vi "VI Tree.vi"   [LabVIEW 2013, in "Keithley 2000.lvlib"]
doc: "This is the instrument driver for the Keithley 2000 Series instruments. The VI Tree displays all the user-callable VIs of the instrument driver in an organized table."
uses:
  Keithley 2000.lvlib
  Configure/Configure Route Single.vi
panel:
  # "© 2003, National Instruments.  All Rights Reserved."
  # "SEE DIAGRAM\nFOR VI TREE."
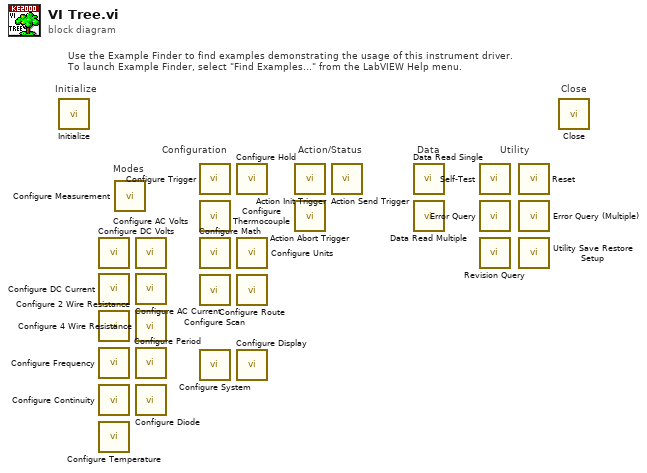
[diagram p0: block diagram]
diagram:
  # "Modes"
  # "Use the Example Finder to find examples demonstrating the usage of this instrument driver.\nTo launch Example Finder, select \"Find Examples...\" from the LabVIEW Help menu."
  # "Configuration"
  # "Utility"
  # "Data"
  # "Action/Status"
  # "Close"
  # "Initialize"
  n1 = call "Initialize.vi"() -> ()  [unwired: 18 in, 2 out]
  n2 = call "Configure DC Volts.vi"() -> ()  [unwired: 18 in, 2 out]
  n3 = call "Configure DC Current.vi"() -> ()  [unwired: 18 in, 2 out]
  n4 = call "Configure 2 Wire Resistance.vi"() -> ()  [unwired: 18 in, 2 out]
  n5 = call "Configure Frequency.vi"() -> ()  [unwired: 18 in, 2 out]
  n6 = call "Configure Continuity.vi"() -> ()  [unwired: 18 in, 2 out]
  n7 = call "Configure Temperature.vi"() -> ()  [unwired: 18 in, 2 out]
  n8 = call-poly "Configure Measurement.vi"() -> ()  [unwired: 18 in, 2 out]
  n9 = call "Configure AC Volts.vi"() -> ()  [unwired: 18 in, 2 out]
  n10 = call "Configure AC Current.vi"() -> ()  [unwired: 18 in, 2 out]
  n11 = call "Configure 4 Wire Resistance.vi"() -> ()  [unwired: 18 in, 2 out]
  n12 = call "Configure Period.vi"() -> ()  [unwired: 18 in, 2 out]
  n13 = call "Configure Diode.vi"() -> ()  [unwired: 18 in, 2 out]
  n14 = call "Configure Trigger.vi"() -> ()  [unwired: 18 in, 2 out]
  n15 = call "Configure Thermocouple.vi"() -> ()  [unwired: 18 in, 2 out]
  n16 = call "Configure Math.vi"() -> ()  [unwired: 18 in, 2 out]
  n17 = call "Configure Scan.vi"() -> ()  [unwired: 18 in, 2 out]
  n18 = call "Configure System.vi"() -> ()  [unwired: 18 in, 2 out]
  n19 = call "Configure Hold.vi"() -> ()  [unwired: 18 in, 2 out]
  n20 = call "Configure Units.vi"() -> ()  [unwired: 18 in, 2 out]
  n21 = call-poly "Configure Route.vi"() -> ()  [unwired: 18 in, 2 out]
  n22 = call "Configure Display.vi"() -> ()  [unwired: 18 in, 2 out]
  n23 = call "Action Init Trigger.vi"() -> ()  [unwired: 18 in, 2 out]
  n24 = call "Action Abort Trigger.vi"() -> ()  [unwired: 18 in, 2 out]
  n25 = call "Action Send Trigger.vi"() -> ()  [unwired: 18 in, 2 out]
  n26 = call "Data Read Single.vi"() -> ()  [unwired: 15 in, 5 out]
  n27 = call "Data Read Multiple.vi"() -> ()  [unwired: 15 in, 5 out]
  n28 = call "Self-Test.vi"() -> ()  [unwired: 16 in, 4 out]
  n29 = call "Error Query.vi"() -> ()  [unwired: 16 in, 4 out]
  n30 = call "Revision Query.vi"() -> ()  [unwired: 16 in, 4 out]
  n31 = call "Reset.vi"() -> ()  [unwired: 18 in, 2 out]
  n32 = call "Error Query (Multiple).vi"() -> ()  [unwired: 16 in, 4 out]
  n33 = call "Utility Save Restore Setup.vi"() -> ()  [unwired: 18 in, 2 out]
  n34 = call "Close.vi"() -> ()  [unwired: 19 in, 1 out]
